vi "顏色轉數字.vi"(3 "顏色數字":dbl) -> (1 "數字":dbl)   [LabVIEW 2014]
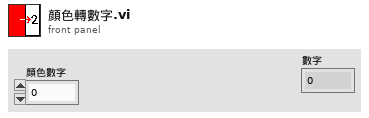
[diagram p1: front panel]
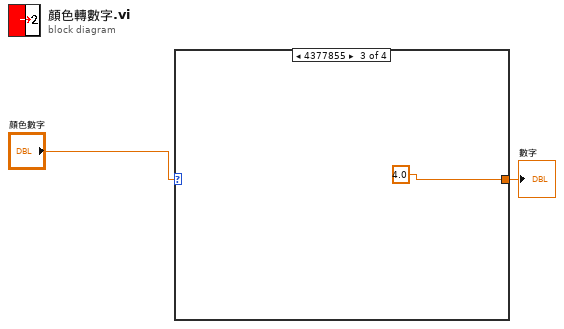
[diagram p0: block diagram]
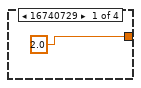
[diagram p2: hidden frame]
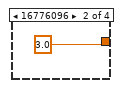
[diagram p3: hidden frame]
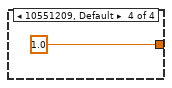
[diagram p4: hidden frame]
diagram:
  n1 = case shown="4377855" "顏色數字" {
    tunnel: [2.0 3.0 4.0 1.0] -> w1
    frame 16740729 {
    }
    frame 16776096 {
    }
    frame 4377855 {
    }
    frame 10551209, Default {
    }
  }
  "數字" <- w1
